vi "Global 5.vi"() -> ()   [LabVIEW 2019]
panel:
  in  "Setpoint":dbl
  in  "temperature":dbl
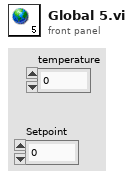
[diagram p1: front panel]
diagram:
